vi "Is Valid (Parent).vi"(8 "error in (no error)":errorcluster, 11 "BlueLogParent in":refnum<class "BlueLogParent_OpenSource.lvclass">) -> (0 "error out":errorcluster, 2 "Is Valid?":bool, 3 "BlueLogParent out":refnum<class "BlueLogParent_OpenSource.lvclass">)   [LabVIEW 2020, in "BlueLogParent_OpenSource.lvclass"]
doc: "This method will return TRUE if the handle is value"
uses:
  BlueLogParent_OpenSource.lvclass
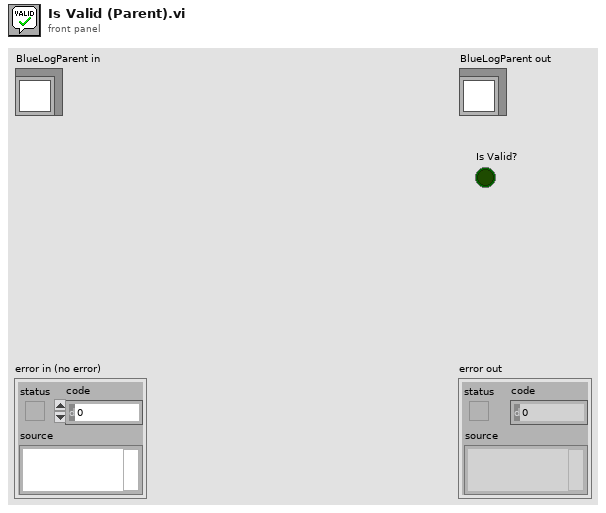
[diagram p1: front panel]
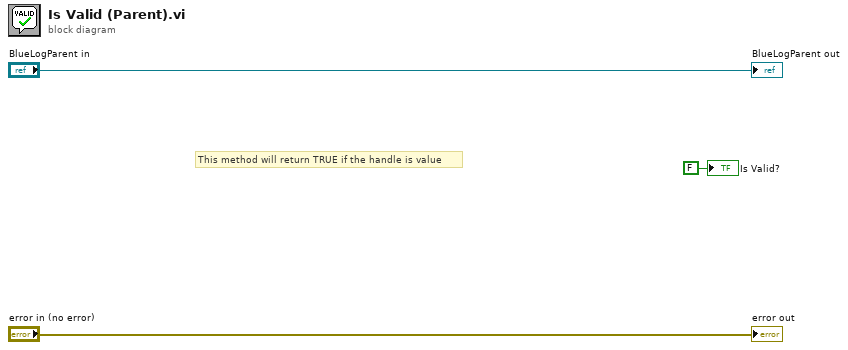
[diagram p0: block diagram]
diagram:
  # "This method will return TRUE if the handle is value"
  "error out" <- "error in (no error)"
  "BlueLogParent out" <- "BlueLogParent in"
  "Is Valid?" <- FALSE ("Is Valid?")
